vi "CallC.vi"(8 "error in (no error)":errorcluster, 10 "Edges":T1, 11 "path to Pix2Pos.exe":path) -> (0 "error out":errorcluster)   [LabVIEW 2022 SP3]
doc: "This VI calls a C programm with a command line\n\nThe command line contains the edges of the table, RGB values of the balls, RGB values of the background and the size of the balls.\nIf the C programm finds errors, the VI \"Error Cluster From Error Code\" write them down in the error cluster.\n\n--/!\\-- WARNING --/!\\-- \n\nThis VI uses predefined RGB ranges to detect each ball:\n\nRed ball :\nR : [91...255]\nG: [0...80]\nB : [0...130]\n\nYellow ball :\nR : [170...255]\nG: [176...255]\nB : [0...175]\n\nWhite ball :\nR : [100...255]\nG: [150...255]\nB : [150...255]\n\nBackground :\nR : [46...63]\nG: [77...93]\nB : [150...185]\n\nBallsize : 13 px\n\n--/!\\-- WARNING --/!\\-- \n\nInputs :\n- The path to Pix2Pos.exe\n- The edges coordinates\n- Error in\n\nOutputs :\n- Error out"
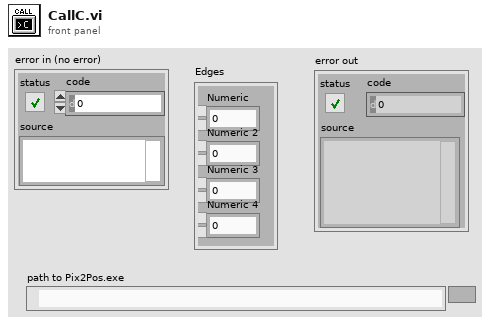
[diagram p1: front panel]
types:
  T1 = cluster{"Numeric":u32, "Numeric 2":u32, "Numeric 3":u32, "Numeric 4":u32}
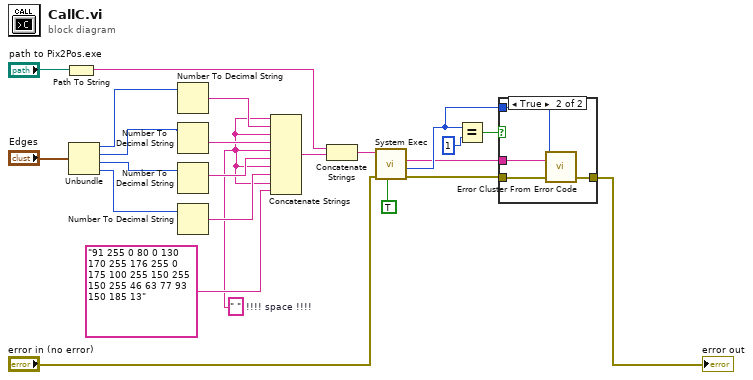
[diagram p0: block diagram]
diagram:
  w8 = " "  # !!!! space !!!!
  n1 = Path To String(path="path to Pix2Pos.exe") -> (string=w10:string)
  n2 = Unbundle("Edges") -> ("Numeric"=w16:u32, "Numeric 2"=w15:u32, "Numeric 3"=w14:u32, "Numeric 4"=w13:u32)
  n3 = Number To Decimal String(number=w16) -> (decimal integer string=w22:string)  [unwired: 1 in]
  n4 = Number To Decimal String(number=w15) -> (decimal integer string=w21:string)  [unwired: 1 in]
  n5 = Number To Decimal String(number=w14) -> (decimal integer string=w20:string)  [unwired: 1 in]
  n6 = Number To Decimal String(number=w13) -> (decimal integer string=w19:string)  [unwired: 1 in]
  n7 = Concatenate Strings(w8, w22, w8, w21, w8, w20, w8, w19, w8, "91 255 0 80 0 130 170 255 176 255 0 175 100 255 150 255 150 255 46 63 77 93 150 185 13") -> (w9:string)
  n8 = Concatenate Strings(w10, w9) -> (w7:string)
  n9 = call <vilib>:"System Exec.vi"("run minimized? (F)"=TRUE, "error in (no error)"="error in (no error)", "command line"=w7) -> ("error out"=w4:errorcluster, "return code"=w3:i32, "standard error"=w2:string)  [unwired: 5 in, 1 out]
  n10 = Equal?(x=w3, y=1) -> (x = y?=w6:bool)
  n11 = case shown="True" w6 {
    tunnel: w2 -> [_ w28]
    tunnel: w3 -> [_ w27]
    tunnel: w4 -> [w24 w26]
    tunnel: [w24 w25] -> w1
    frame False {
    }
    frame True {
      n12 = call <vilib>:"Error Cluster From Error Code.vi"("error in (no error)"=w26, "error message (\"\")"=w28, "error code (0)"=w27) -> ("error out"=w25:errorcluster)  [unwired: 6 in]
    }
  }
  "error out" <- w1
